vi "Instrument Manager Loop.vi"(8 "System Control":refnum<queue>, 11 "Instrument Manager":refnum<queue>) -> (0 "error out":errorcluster)   [LabVIEW 2020, in "ChromTech Next Gen Pump.lvlib" / "Instrument Manager.lvlib"]
uses:
  Instrument Manager/Instrument Manager.lvlib
  support/Message Queue/Message Cluster.ctl
  Instrument Manager/Instrument State.ctl
  <vilib>/Utility/error.llb/Error Cluster From Error Code.vi
  <vilib>/ErrorRing/Error Ring.xnode
  support/Message Queue/Message Queue.lvlib
  ChromTech Next Gen Pump.lvlib
  <instrlib>/RxnRover/ChromtechNextGenDriver/ChromTech MX-Class Drivers.lvlib
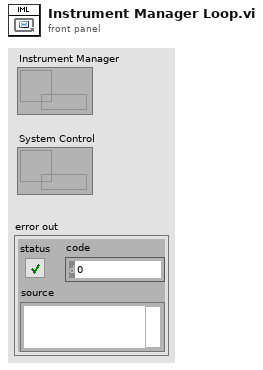
[diagram p1: front panel]
types:
  T1 = typedef "ChromTech Next Gen Pump.lvlib/Instrument Manager.lvlib/Instrument State.ctl" = cluster{"VISA Resource":refnum<visa-resource-name>, "Flow Rate":dbl, "Running":bool, "Running Since":timestamp, "Pressure Data Point":cluster{"Time Stamp":timestamp, "Value":dbl}, "Upper Pressure Fault":bool, "Lower Pressure Fault":bool, "Motor Stall Fault":bool, "Sampling Rate (sec/sample)":dbl, "Retry Attempts":i32, "Fast Comms":bool}
  T2 = cluster{"seconds since 1Jan1904":timestamp, "Pressure":dbl}
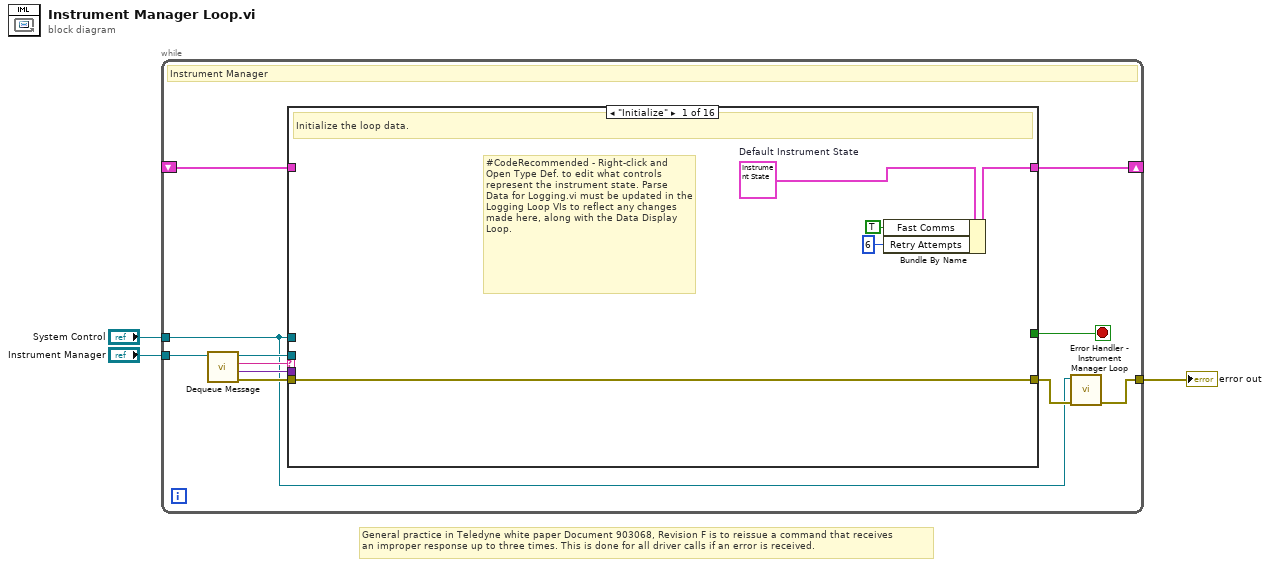
[diagram p0: block diagram]
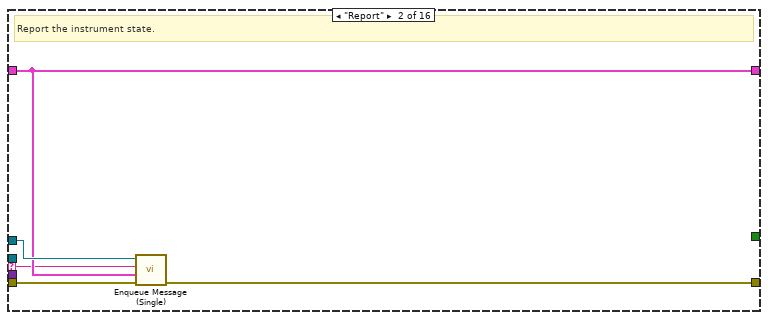
[diagram p2: hidden frame]
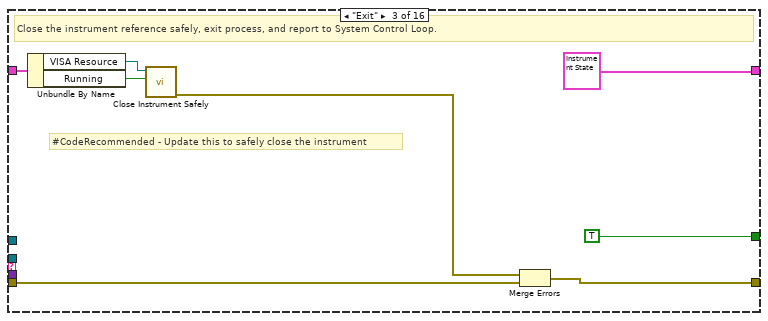
[diagram p3: hidden frame]
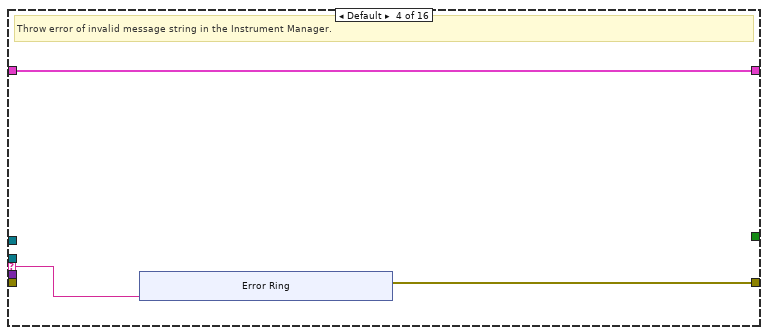
[diagram p4: hidden frame]
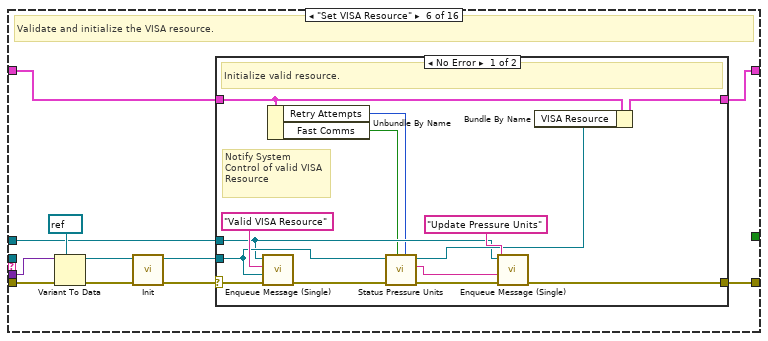
[diagram p6: hidden frame]
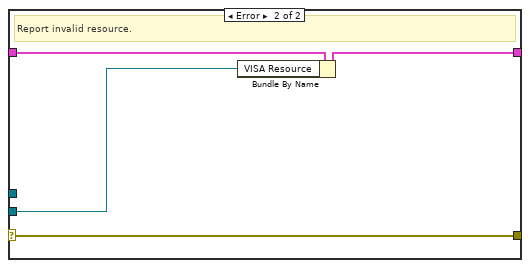
[diagram p7: hidden frame]
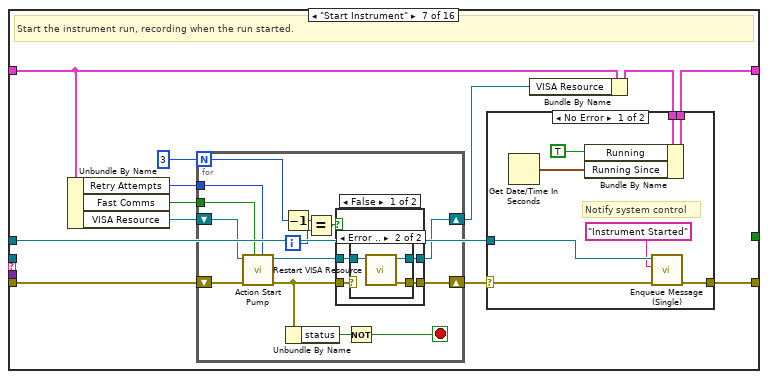
[diagram p8: hidden frame]
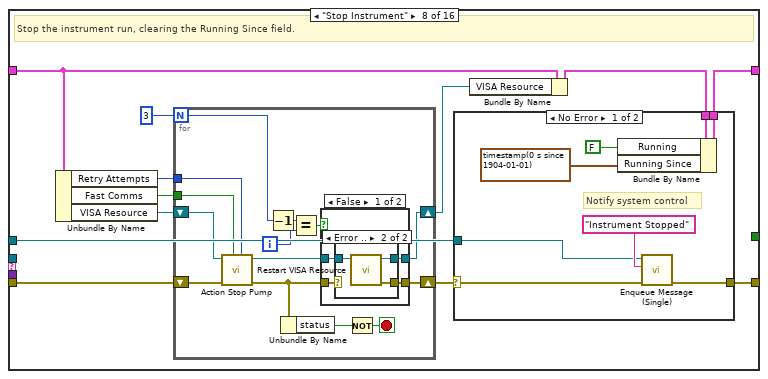
[diagram p12: hidden frame]
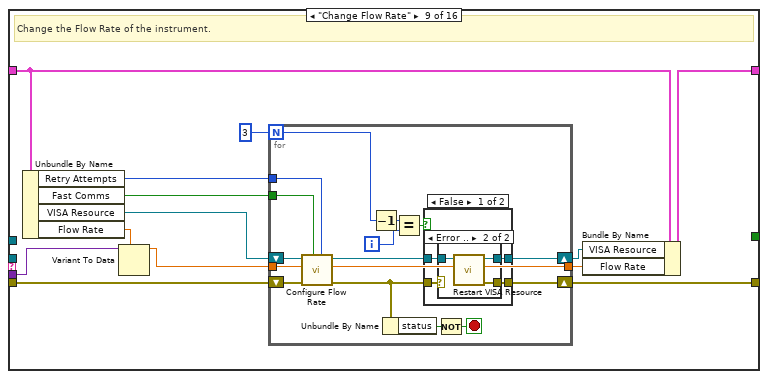
[diagram p16: hidden frame]
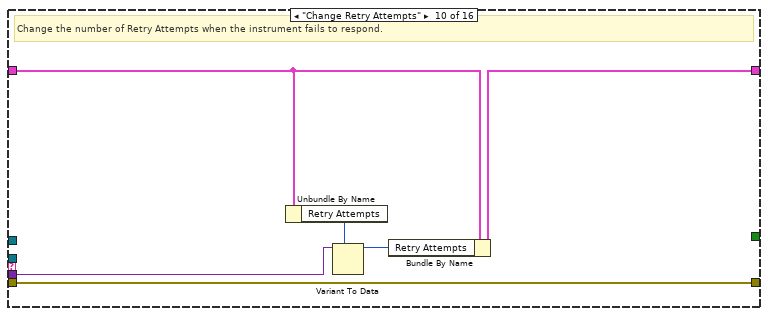
[diagram p19: hidden frame]
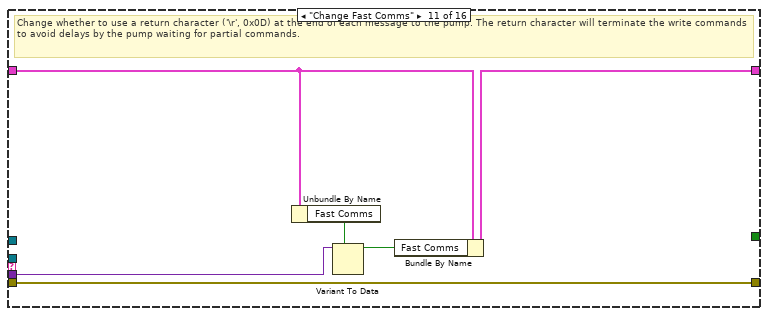
[diagram p20: hidden frame]
diagram:
  # "General practice in Teledyne white paper Document 903068, Revision F is to reissue a command that receives\nan improper response up to three times. This is done for all driver calls if an error is received."
  n1 = while {
    tunnel: "Instrument Manager" -> [w14]
    tunnel: "System Control" -> [w4]
    tunnel: [w8] -> w1
    shift-right: [w6] -> _
    shift-left: _ -> [w7]
    stop <- w5 stop-if-true
    # "Instrument Manager"
    n2 = call "Dequeue Message.vi"("Message Queue"=w14) -> ("error out"=w10:errorcluster, "Message Data"=w11:variant, "Message"=w13:string, "dup Message Queue"=w12:refnum<queue>)  [unwired: 7 in]
    n3 = case shown="\"Initialize\"" w13 {
      selector: w13 -> [_ w20 _ w34 _ _ _ _ _ _ _ _ _ _ _ _]
      tunnel: w12 -> [_ _ _ _ _ _ _ _ _ _ _ _ _ _ _ _]
      tunnel: w4 -> [_ w23 _ _ _ w45 w84 w131 _ _ _ _ _ _ _ _]
      tunnel: w11 -> [_ _ _ _ _ w52 _ _ w179 w212 w218 _ _ _ _ _]
      tunnel: w10 -> [w18 w24 w27 _ w43 w51 w82 w129 w174 w209 w215 w222 w231 w266 w306 w347]
      tunnel: [w18 w22 w26 w33 w43 w55 w85 w132 w173 w209 w215 w222 w230 w265 w304 w340] -> w9
      tunnel: w7 -> [_ w21 w32 w35 w44 w54 w81 w127 w178 w211 w217 w221 w229 w267 w303 w344]
      tunnel: [w17 w21 T1 {"VISA Resource"="", "Flow Rate"=0.0, "Running"=FALSE, "Running Since"=timestamp(0 s since 1904-01-01), "Pressure Data Point"={"Time Stamp"=timestamp(0 s since 1904-01-01), "Value"=0.0}, "Upper Pressure Fault"=FALSE, "Lower Pressure Fault"=FALSE, "Motor Stall Fault"=FALSE, "Sampling Rate (sec/sample)"=0.0, "Retry Attempts"=0, "Fast Comms"=FALSE} w35 w44 w53 w83 w130 w180 w213 w219 w221 w232 w270 w305 w346] -> w6
      tunnel: [_ _ TRUE _ _ _ _ _ _ _ _ _ _ _ _ _] -> w5
      frame "Initialize" {
        w19 = T1 {"VISA Resource"="", "Flow Rate"=0.0, "Running"=FALSE, "Running Since"=timestamp(0 s since 1904-01-01), "Pressure Data Point"={"Time Stamp"=timestamp(0 s since 1904-01-01), "Value"=0.0}, "Upper Pressure Fault"=FALSE, "Lower Pressure Fault"=FALSE, "Motor Stall Fault"=FALSE, "Sampling Rate (sec/sample)"=0.0, "Retry Attempts"=0, "Fast Comms"=FALSE}  # Default Instrument State
        # "#CodeRecommended - Right-click and Open Type Def. to edit what controls represent the instrument state. Parse Data for Logging.vi must be updated in the Logging Loop VIs to reflect any changes made here, along with the Data Display Loop."
        # "Initialize the loop data."
        n4 = Bundle By Name(cluster=w19, "Fast Comms"=TRUE, "Retry Attempts"=6) -> (w17:T1)
      }
      frame "Report" {
        # "Report the instrument state."
        n5 = call "Enqueue Message (Single).vi"("error in (no error)"=w24, "Message Data"=w21, "Message"=w20, "Message Queue"=w23) -> ("error out"=w22:errorcluster)  [unwired: 6 in, 1 out]
      }
      frame "Exit" {
        # "#CodeRecommended - Update this to safely close the instrument"
        # "Close the instrument reference safely, exit process, and report to System Control Loop."
        n6 = Unbundle By Name(w32) -> ("VISA Resource"=w30:refnum<visa-resource-name>, "Running"=w31:bool)
        n7 = call "Close Instrument Safely.vi"("Running (F)"=w31, "VISA Refnum in"=w30) -> ("error out"=w25:errorcluster)  [unwired: 9 in]
        n8 = Merge Errors(w25, w27) -> (w26:errorcluster)
      }
      frame Default {
        # "Throw error of invalid message string in the Instrument Manager."
        n9 = xnode "Error Ring"("parameter 0"=w34) -> ("error out"=w33:errorcluster)
      }
      frame "--- Copy This Frame ---" {
        # "Copy this frame and add responses to instrument specific messages."
      }
      frame "Set VISA Resource" {
        # "Validate and initialize the VISA resource."
        n10 = Variant To Data(error in=w51, type=refnum<visa-resource-name> refnum, Variant=w52) -> (data=w49:refnum<visa-resource-name>, error out=w50:errorcluster)
        n11 = call "Init.vi"("error in (no error)"=w50, "VISA resource in"=w49) -> ("error out"=w46:errorcluster, "VISA resource out"=w47:refnum<visa-resource-name>)  [unwired: 8 in]
        n12 = case shown="No Error" w46 {
          selector: w46 -> [w69 w70]
          tunnel: w47 -> [w62 w71]
          tunnel: [w64 w70] -> w55
          tunnel: w54 -> [w58 w73]
          tunnel: [w67 w72] -> w53
          tunnel: w45 -> [w60 _]
          frame No Error {
            # "Notify System Control of valid VISA Resource"
            # "Initialize valid resource."
            n13 = call "Enqueue Message (Single).vi"("error in (no error)"=w69, "Message Data"=w62, "Message"="Valid VISA Resource", "Message Queue"=w60) -> ("error out"=w66:errorcluster)  [unwired: 6 in, 1 out]
            n14 = Unbundle By Name(w58) -> ("Retry Attempts"=w57:i32, "Fast Comms"=w56:bool)
            n15 = call <instrlib>:"Status Pressure Units.vi"("Retry Attempts (0)"=w57, "Fast Comms (F)"=w56, "error in (no error)"=w66, "VISA resource name"=w62) -> ("error out"=w65:errorcluster, "Pressure Units"=w59:string, "VISA resource name out"=w61:refnum<visa-resource-name>)  [unwired: 5 in]
            n16 = call "Enqueue Message (Single).vi"("error in (no error)"=w65, "Message Data"=w59, "Message"="Update Pressure Units", "Message Queue"=w60) -> ("error out"=w64:errorcluster)  [unwired: 6 in, 1 out]
            n17 = Bundle By Name(cluster=w58, "VISA Resource"=w61) -> (w67:T1)
          }
          frame Error {
            # "Report invalid resource."
            n18 = Bundle By Name(cluster=w73, "VISA Resource"=w71) -> (w72:T1)
          }
        }
      }
      frame "Start Instrument" {
        # "Start the instrument run, recording when the run started."
        n19 = Unbundle By Name(w81) -> ("Retry Attempts"=w77:i32, "Fast Comms"=w78:bool, "VISA Resource"=w80:refnum<visa-resource-name>)
        n20 = for {
          N: 3 -> [w89]
          tunnel: w78 -> [w97]
          tunnel: w77 -> [w96]
          shift-right: [w86] -> w79
          shift-left: w82 -> [w99]
          shift-right: [w90] -> w74
          shift-left: w80 -> [w98]
          i -> [w88]
          stop <- w94 stop-if-true
          n21 = call <instrlib>:"Action Start Pump.vi"("Retry Attempts (0)"=w96, "Fast Comms (F)"=w97, "error in"=w99, "VISA resource name"=w98) -> ("error out"=w87:errorcluster, "VISA resource name out"=w91:refnum<visa-resource-name>)  [unwired: 6 in]
          n22 = Decrement(x=w89) -> (x-1=w93:i32)
          n23 = Unbundle By Name(w87) -> ("status"=w95:bool)
          n24 = Equal?(x=w93, y=w88) -> (x = y?=w92:bool)
          n25 = case shown="False" w92 {
            tunnel: [w103 w110] -> w86
            tunnel: w91 -> [w102 w109]
            tunnel: w87 -> [w101 w110]
            tunnel: [w100 w109] -> w90
            frame False {
              n26 = case shown="Error .." w101 {
                selector: w101 -> [w105 _]
                tunnel: [w105 w108] -> w103
                tunnel: w102 -> [w104 w107]
                tunnel: [w104 w106] -> w100
                frame No Error {
                }
                frame Error {
                  n27 = call "Restart VISA Resource.vi"("VISA Refnum in"=w107) -> ("error out"=w108:errorcluster, "VISA resource name out"=w106:refnum<visa-resource-name>)  [unwired: 9 in]
                }
              }
            }
            frame True {
            }
          }
          n28 = Not(x=w95) -> (.not. x?=w94:bool)
        }
        n29 = Bundle By Name(cluster=w81, "VISA Resource"=w74) -> (w75:T1)
        n30 = case shown="No Error" w79 {
          selector: w79 -> [w111 w120]
          tunnel: [w118 w120] -> w85
          tunnel: w84 -> [w117 _]
          tunnel: [w115 w119] -> w83
          tunnel: w75 -> [w112 w119]
          frame No Error {
            # "Notify system control"
            n31 = Get Date/Time In Seconds() -> (seconds since 1Jan1904=w113:timestamp)
            n32 = Bundle By Name(cluster=w112, "Running"=TRUE, "Running Since"=w113) -> (w115:T1)
            n33 = call "Enqueue Message (Single).vi"("error in (no error)"=w111, "Message"="Instrument Started", "Message Queue"=w117) -> ("error out"=w118:errorcluster)  [unwired: 7 in, 1 out]
          }
          frame Error {
          }
        }
      }
      frame "Stop Instrument" {
        # "Stop the instrument run, clearing the Running Since field."
        n34 = Unbundle By Name(w127) -> ("Retry Attempts"=w124:i32, "Fast Comms"=w125:bool, "VISA Resource"=w126:refnum<visa-resource-name>)
        n35 = for {
          N: 3 -> [w135]
          tunnel: w125 -> [w144]
          tunnel: w124 -> [w143]
          shift-right: [w136] -> w128
          shift-left: w129 -> [w146]
          shift-right: [w138] -> w121
          shift-left: w126 -> [w145]
          i -> [w134]
          stop <- w141 stop-if-true
          n36 = call <instrlib>:"Action Stop Pump.vi"("Retry Attempts (0)"=w143, "Fast Comms (F)"=w144, "error in"=w146, "VISA resource name"=w145) -> ("error out"=w137:errorcluster, "VISA resource name out"=w139:refnum<visa-resource-name>)  [unwired: 6 in]
          n37 = Decrement(x=w135) -> (x-1=w140:i32)
          n38 = Unbundle By Name(w137) -> ("status"=w142:bool)
          n39 = Equal?(x=w140, y=w134) -> (x = y?=w133:bool)
          n40 = case shown="False" w133 {
            tunnel: [w150 w157] -> w136
            tunnel: w139 -> [w149 w156]
            tunnel: w137 -> [w148 w157]
            tunnel: [w147 w156] -> w138
            frame False {
              n41 = case shown="Error .." w148 {
                selector: w148 -> [w152 _]
                tunnel: [w152 w155] -> w150
                tunnel: w149 -> [w151 w154]
                tunnel: [w151 w153] -> w147
                frame No Error {
                }
                frame Error {
                  n42 = call "Restart VISA Resource.vi"("VISA Refnum in"=w154) -> ("error out"=w155:errorcluster, "VISA resource name out"=w153:refnum<visa-resource-name>)  [unwired: 9 in]
                }
              }
            }
            frame True {
            }
          }
          n43 = Not(x=w142) -> (.not. x?=w141:bool)
        }
        n44 = Bundle By Name(cluster=w127, "VISA Resource"=w121) -> (w122:T1)
        n45 = case shown="No Error" w128 {
          selector: w128 -> [w158 w167]
          tunnel: w122 -> [w165 w166]
          tunnel: [w164 w167] -> w132
          tunnel: w131 -> [w162 _]
          tunnel: [w161 w166] -> w130
          frame No Error {
            # "Notify system control"
            n46 = Bundle By Name(cluster=w165, "Running"=FALSE, "Running Since"=timestamp(0 s since 1904-01-01)) -> (w161:T1)
            n47 = call "Enqueue Message (Single).vi"("error in (no error)"=w158, "Message"="Instrument Stopped", "Message Queue"=w162) -> ("error out"=w164:errorcluster)  [unwired: 7 in, 1 out]
          }
          frame Error {
          }
        }
      }
      frame "Change Flow Rate" {
        # "Change the Flow Rate of the instrument."
        n48 = Unbundle By Name(w178) -> ("Retry Attempts"=w171:i32, "Fast Comms"=w170:bool, "VISA Resource"=w176:refnum<visa-resource-name>, "Flow Rate"=w177:dbl)
        n49 = Variant To Data(type=w177, Variant=w179) -> (data=w175:dbl)  [unwired: 1 in, 1 out]
        n50 = for {
          N: 3 -> [w183]
          tunnel: w175 -> [w195]
          tunnel: [w194] -> w172
          tunnel: w171 -> [w193]
          tunnel: w170 -> [w192]
          shift-right: [w186] -> w173
          shift-left: w174 -> [w191]
          shift-right: [w184] -> w168
          shift-left: w176 -> [w196]
          i -> [w182]
          stop <- w189 stop-if-true
          n51 = call <instrlib>:"Configure Flow Rate.vi"("Retry Attempts (0)"=w193, "Fast Comms (F)"=w192, "error in"=w191, "Flow Input (ml/min)"=w195, "VISA resource name"=w196) -> ("error out"=w187:errorcluster, "Flow Output"=w194:dbl, "VISA resource name out"=w185:refnum<visa-resource-name>)  [unwired: 4 in]
          n52 = Decrement(x=w183) -> (x-1=w188:i32)
          n53 = Unbundle By Name(w187) -> ("status"=w190:bool)
          n54 = Equal?(x=w188, y=w182) -> (x = y?=w181:bool)
          n55 = case shown="False" w181 {
            tunnel: [w200 w207] -> w186
            tunnel: w185 -> [w199 w206]
            tunnel: w187 -> [w198 w207]
            tunnel: [w197 w206] -> w184
            frame False {
              n56 = case shown="Error .." w198 {
                selector: w198 -> [w202 _]
                tunnel: [w202 w205] -> w200
                tunnel: w199 -> [w201 w204]
                tunnel: [w201 w203] -> w197
                frame No Error {
                }
                frame Error {
                  n57 = call "Restart VISA Resource.vi"("VISA Refnum in"=w204) -> ("error out"=w205:errorcluster, "VISA resource name out"=w203:refnum<visa-resource-name>)  [unwired: 9 in]
                }
              }
            }
            frame True {
            }
          }
          n58 = Not(x=w190) -> (.not. x?=w189:bool)
        }
        n59 = Bundle By Name(cluster=w178, "VISA Resource"=w168, "Flow Rate"=w172) -> (w180:T1)
      }
      frame "Change Retry Attempts" {
        # "Change the number of Retry Attempts when the instrument fails to respond."
        n60 = Unbundle By Name(w211) -> ("Retry Attempts"=w208:i32)
        n61 = Variant To Data(type=w208, Variant=w212) -> (data=w210:i32)  [unwired: 1 in, 1 out]
        n62 = Bundle By Name(cluster=w211, "Retry Attempts"=w210) -> (w213:T1)
      }
      frame "Change Fast Comms" {
        # "Change whether to use a return character ('\\r', 0x0D) at the end of each message to the pump. The return character will terminate the write commands to avoid delays by the pump waiting for partial commands."
        n63 = Unbundle By Name(w217) -> ("Fast Comms"=w214:bool)
        n64 = Variant To Data(type=w214, Variant=w218) -> (data=w216:bool)  [unwired: 1 in, 1 out]
        n65 = Bundle By Name(cluster=w217, "Fast Comms"=w216) -> (w219:T1)
      }
      frame "--- Copy for Get State Messages ---" {
        # "Wait 100 ms because if two commands are sent in quick succession, the second will fail."
        # "#CodeNeeded - Use the Bundle by Name function to bundle the new state value into the Instrument State cluster."
        # "#CodeNeeded - Add instrument driver call to query the instrument state requested"
        # "Duplicate this case for messages cases that will query the instrument state."
        n66 = Wait (ms)(milliseconds to wait=u32 100) -> ()  [unwired: 1 out]
      }
      frame "Run State" {
        # "Query the run state of the instrument."
        n67 = Unbundle By Name(w229) -> ("Retry Attempts"=w226:i32, "Fast Comms"=w225:bool, "VISA Resource"=w228:refnum<visa-resource-name>)
        n68 = for {
          N: 3 -> [w234]
          tunnel: [w246] -> w227
          tunnel: w226 -> [w245]
          tunnel: w225 -> [w244]
          shift-right: [w238] -> w230
          shift-left: w231 -> [w243]
          shift-right: [w236] -> w223
          shift-left: w228 -> [w247]
          i -> [w235]
          stop <- w241 stop-if-true
          n69 = call <instrlib>:"Status Run State.vi"("Retry Attempts (0)"=w245, "Fast Comms (F)"=w244, "error in (no error)"=w243, "VISA resource name"=w247) -> ("error out"=w239:errorcluster, "Running?"=w246:bool, "VISA resource name out"=w237:refnum<visa-resource-name>)  [unwired: 5 in]
          n70 = Decrement(x=w234) -> (x-1=w240:i32)
          n71 = Unbundle By Name(w239) -> ("status"=w242:bool)
          n72 = Equal?(x=w240, y=w235) -> (x = y?=w233:bool)
          n73 = case shown="False" w233 {
            tunnel: [w251 w258] -> w238
            tunnel: w237 -> [w250 w257]
            tunnel: w239 -> [w249 w258]
            tunnel: [w248 w257] -> w236
            frame False {
              n74 = case shown="Error .." w249 {
                selector: w249 -> [w253 _]
                tunnel: [w253 w256] -> w251
                tunnel: w250 -> [w252 w255]
                tunnel: [w252 w254] -> w248
                frame No Error {
                }
                frame Error {
                  n75 = call "Restart VISA Resource.vi"("VISA Refnum in"=w255) -> ("error out"=w256:errorcluster, "VISA resource name out"=w254:refnum<visa-resource-name>)  [unwired: 9 in]
                }
              }
            }
            frame True {
            }
          }
          n76 = Not(x=w242) -> (.not. x?=w241:bool)
        }
        n77 = Bundle By Name(cluster=w229, "VISA Resource"=w223, "Running"=w227) -> (w232:T1)
      }
      frame "Pressure" {
        # "Query the pressure value of the instrument."
        n78 = Unbundle By Name(w267) -> ("Retry Attempts"=w261:i32, "Fast Comms"=w262:bool, "VISA Resource"=w264:refnum<visa-resource-name>)
        n79 = for {
          N: 3 -> [w272]
          tunnel: [w284] -> w263
          tunnel: w262 -> [w283]
          tunnel: w261 -> [w282]
          shift-right: [w276] -> w265
          shift-left: w266 -> [w281]
          shift-right: [w274] -> w259
          shift-left: w264 -> [w285]
          i -> [w273]
          stop <- w279 stop-if-true
          n80 = call <instrlib>:"Status Get Pressure.vi"("Retry Attempts (0)"=w282, "Fast Comms (F)"=w283, "error in"=w281, "VISA resource name"=w285) -> ("error out"=w277:errorcluster, "Pressure"=w284:dbl, "VISA resource name out"=w275:refnum<visa-resource-name>)  [unwired: 5 in]
          n81 = Decrement(x=w272) -> (x-1=w278:i32)
          n82 = Unbundle By Name(w277) -> ("status"=w280:bool)
          n83 = Equal?(x=w278, y=w273) -> (x = y?=w271:bool)
          n84 = case shown="False" w271 {
            tunnel: [w289 w296] -> w276
            tunnel: w275 -> [w288 w295]
            tunnel: w277 -> [w287 w296]
            tunnel: [w286 w295] -> w274
            frame False {
              n85 = case shown="Error .." w287 {
                selector: w287 -> [w291 _]
                tunnel: [w291 w294] -> w289
                tunnel: w288 -> [w290 w293]
                tunnel: [w290 w292] -> w286
                frame No Error {
                }
                frame Error {
                  n86 = call "Restart VISA Resource.vi"("VISA Refnum in"=w293) -> ("error out"=w294:errorcluster, "VISA resource name out"=w292:refnum<visa-resource-name>)  [unwired: 9 in]
                }
              }
            }
            frame True {
            }
          }
          n87 = Not(x=w280) -> (.not. x?=w279:bool)
        }
        n88 = Get Date/Time In Seconds() -> (seconds since 1Jan1904=w269:timestamp)
        n89 = Bundle("seconds since 1Jan1904"=w269, "Pressure"=w263) -> (w268:T2)  [unwired: 1 in]
        n90 = Bundle By Name(cluster=w267, "Pressure Data Point"=w268, "VISA Resource"=w259) -> (w270:T1)
      }
      frame "Flow Rate" {
        # "Query the flow rate of the instrument."
        n91 = Unbundle By Name(w303) -> ("Retry Attempts"=w300:i32, "Fast Comms"=w299:bool, "VISA Resource"=w302:refnum<visa-resource-name>)
        n92 = for {
          N: 3 -> [w310]
          tunnel: [w320] -> w301
          tunnel: w300 -> [w319]
          tunnel: w299 -> [w318]
          shift-right: [w312] -> w304
          shift-left: w306 -> [w317]
          shift-right: [w307] -> w297
          shift-left: w302 -> [w321]
          i -> [w309]
          stop <- w315 stop-if-true
          n93 = call <instrlib>:"Status Get Flow Rate.vi"("Retry Attempts (0)"=w319, "Fast Comms (F)"=w318, "error in"=w317, "VISA resource name"=w321) -> ("error out"=w313:errorcluster, "Flow Rate"=w320:dbl, "VISA resource name out"=w308:refnum<visa-resource-name>)  [unwired: 5 in]
          n94 = Unbundle By Name(w313) -> ("status"=w316:bool)
          n95 = Decrement(x=w310) -> (x-1=w314:i32)
          n96 = Equal?(x=w314, y=w309) -> (x = y?=w311:bool)
          n97 = case shown="False" w311 {
            tunnel: [w325 w332] -> w312
            tunnel: w308 -> [w324 w331]
            tunnel: w313 -> [w323 w332]
            tunnel: [w322 w331] -> w307
            frame False {
              n98 = case shown="Error .." w323 {
                selector: w323 -> [w327 _]
                tunnel: [w327 w330] -> w325
                tunnel: w324 -> [w326 w329]
                tunnel: [w326 w328] -> w322
                frame No Error {
                }
                frame Error {
                  n99 = call "Restart VISA Resource.vi"("VISA Refnum in"=w329) -> ("error out"=w330:errorcluster, "VISA resource name out"=w328:refnum<visa-resource-name>)  [unwired: 9 in]
                }
              }
            }
            frame True {
            }
          }
          n100 = Not(x=w316) -> (.not. x?=w315:bool)
        }
        n101 = Bundle By Name(cluster=w303, "VISA Resource"=w297, "Flow Rate"=w301) -> (w305:T1)
      }
      frame "Faults" {
        # "Query the fault status of the instrument."
        n102 = Unbundle By Name(w344) -> ("Retry Attempts"=w336:i32, "Fast Comms"=w335:bool, "VISA Resource"=w343:refnum<visa-resource-name>)
        n103 = for {
          N: 3 -> [w350]
          tunnel: [w362] -> w342
          tunnel: [w361] -> w341
          tunnel: [w360] -> w337
          tunnel: w336 -> [w359]
          tunnel: w335 -> [w358]
          shift-right: [w353] -> w345
          shift-left: w347 -> [w364]
          shift-right: [w351] -> w333
          shift-left: w343 -> [w363]
          i -> [w349]
          stop <- w356 stop-if-true
          n104 = call <instrlib>:"Status Faults.vi"("VISA resource name"=w363, "Fast Comms (F)"=w358, "Retry Attempts (0)"=w359, "error in (no error)"=w364) -> ("VISA resource name out"=w352:refnum<visa-resource-name>, "Upper Pressure Fault"=w361:bool, "Lower Pressure Fault"=w362:bool, "Motor Stall Fault"=w360:bool, "error out"=w354:errorcluster)  [unwired: 7 in]
          n105 = Decrement(x=w350) -> (x-1=w355:i32)
          n106 = Unbundle By Name(w354) -> ("status"=w357:bool)
          n107 = Equal?(x=w355, y=w349) -> (x = y?=w348:bool)
          n108 = Not(x=w357) -> (.not. x?=w356:bool)
          n109 = case shown="False" w348 {
            tunnel: [w368 w375] -> w353
            tunnel: w352 -> [w367 w374]
            tunnel: w354 -> [w366 w375]
            tunnel: [w365 w374] -> w351
            frame False {
              n110 = case shown="Error .." w366 {
                selector: w366 -> [w370 _]
                tunnel: [w370 w373] -> w368
                tunnel: w367 -> [w369 w372]
                tunnel: [w369 w371] -> w365
                frame No Error {
                }
                frame Error {
                  n111 = call "Restart VISA Resource.vi"("VISA Refnum in"=w372) -> ("error out"=w373:errorcluster, "VISA resource name out"=w371:refnum<visa-resource-name>)  [unwired: 9 in]
                }
              }
            }
            frame True {
            }
          }
        }
        n112 = Build Array(w337, w342, w341) -> (w338:bool[])
        n113 = Bundle By Name(cluster=w344, "VISA Resource"=w333, "Upper Pressure Fault"=w341, "Lower Pressure Fault"=w342, "Motor Stall Fault"=w337) -> (w346:T1)
        n114 = Or Array Elements(Boolean array=w338) -> (logical OR=w339:bool)
        n115 = case shown="True" w339 {
          tunnel: w345 -> [w376 w380]
          tunnel: [w376 w379] -> w340
          tunnel: w338 -> [_ w377]
          frame False {
          }
          frame True {
            n116 = call "Error Cluster from Fault.vi"("Fault indicators"=w377) -> ("error out"=w378:errorcluster)  [unwired: 10 in]
            n117 = Merge Errors(w378, w380) -> (w379:errorcluster)
          }
        }
      }
    }
    n118 = call "Error Handler - Instrument Manager Loop.vi"("error in (no error)"=w9, "Message Queue"=w4) -> ("dup error in"=w8:errorcluster)  [unwired: 8 in, 1 out]
  }
  "error out" <- w1
